vi "Array processor.vi"(10 "Source array":bool[][](array[boolean]), 11 "Pixel size":dbl=12.19 step=0.01) -> (0 "Lenght array":dbl[][](array[numeric]), 3 "T/F product array":bool[][](array[boolean]))   [LabVIEW 2016]
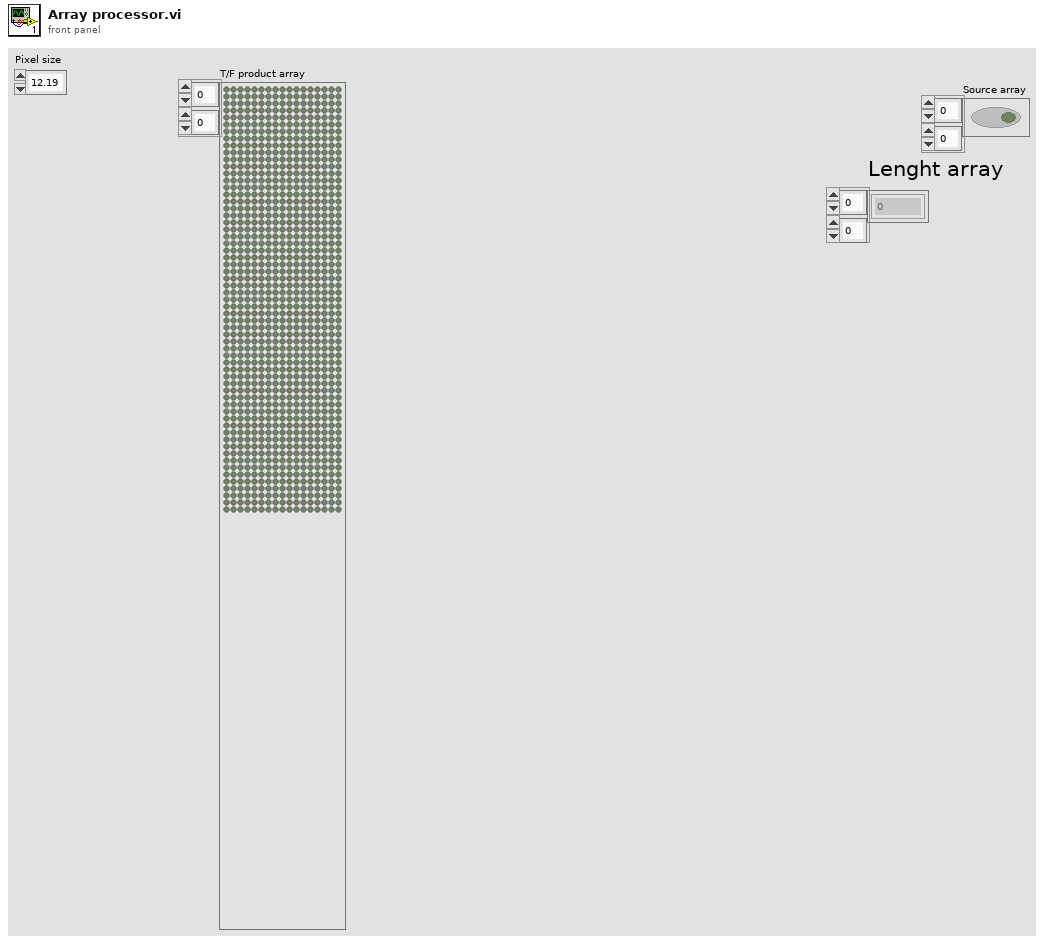
[diagram p1: front panel]
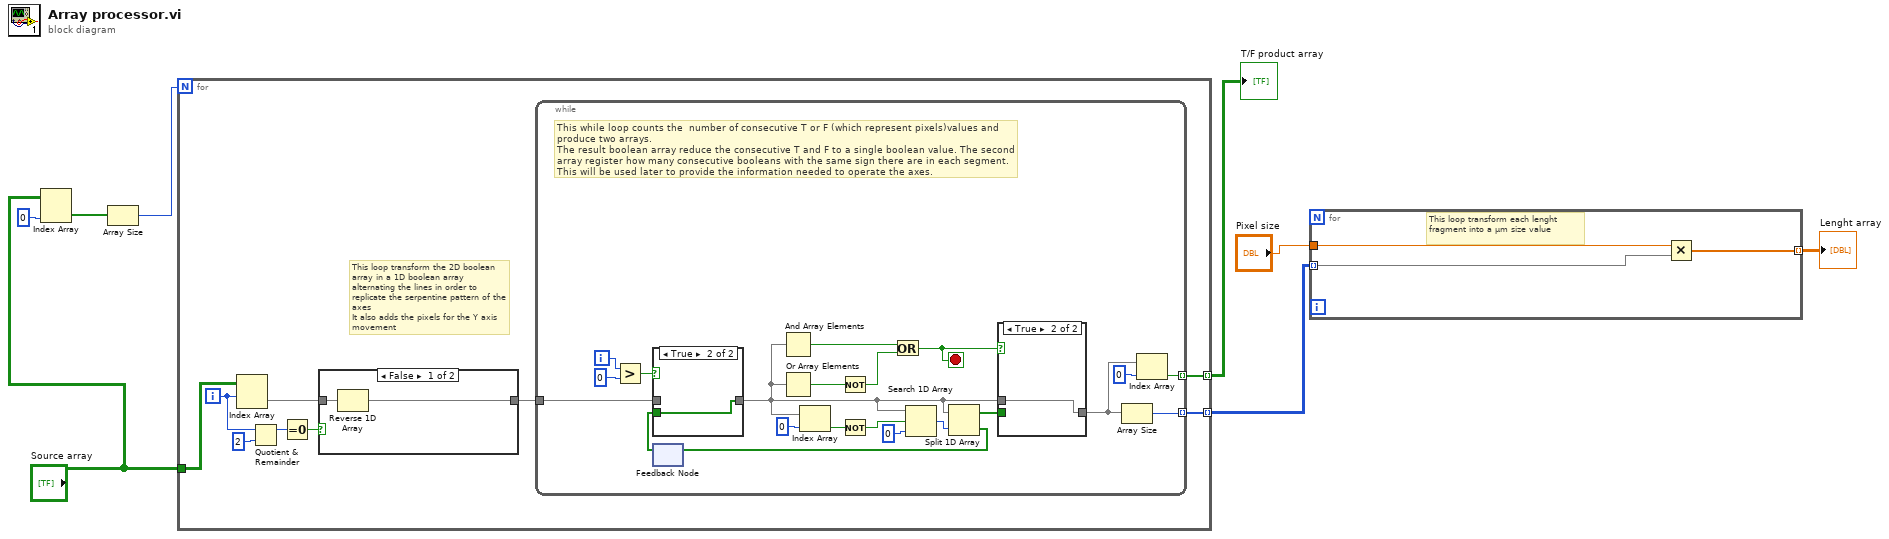
[diagram p0: block diagram]
diagram:
  n1 = Index Array(array="Source array", index (col)=0 ("disabled index (col)")) -> (element=w6:bool[])  [unwired: 1 in]
  n2 = Array Size(array=w6) -> (size(s)=w4:i32)
  n3 = for {
    N: w4 -> [_]
    tunnel: "Source array" -> [w12]
    tunnel: [w10] -> w3 mode=indexing
    tunnel: [w9] -> w8 mode=indexing
    i -> [w15]
    # "This loop transform the 2D boolean array in a 1D boolean array alternating the lines in order to replicate the serpentine pattern of the axes\nIt also adds the pixels for the Y axis movement"
    n4 = Index Array(array=w12, index (row)=w15) -> (element=w13:bool[])  [unwired: 1 in]
    n5 = Quotient & Remainder(x=w15, y=2) -> (x-y*floor(x/y)=w17:i32)  [unwired: 1 out]
    n6 = Equal To 0?(x=w17) -> (x = 0?=w14:bool)
    n7 = case shown="False" w14 {
      tunnel: w13 -> [w44 w45]
      tunnel: [w43 w45] -> w11
      frame False {
        n8 = Reverse 1D Array(array=w44) -> (reversed array=w43:bool[])
      }
      frame True {
      }
    }
    n9 = while {
      tunnel: w11 -> [w32]
      tunnel: [w37] -> w10 mode=indexing
      tunnel: [w18] -> w9 mode=indexing
      i -> [w29]
      stop <- w21 stop-if-true
      # "This while loop counts the  number of consecutive T or F (which represent pixels)values and produce two arrays.\nThe result boolean array reduce the consecutive T and F to a single boolean value. The second array register how many consecutive booleans with the same sign there are in each segment. This will be used later to provide the information needed to operate the axes."
      n10 = Greater?(x=w29, y=0) -> (0:w30:bool)
      n11 = feedback #1() -> (w31:bool[])  [unwired: 1 in]
      n12 = case shown="True" w30 {
        tunnel: w32 -> [w41 _]
        tunnel: [w41 w42] -> w22
        tunnel: w31 -> [_ w42]
        frame False {
        }
        frame True {
        }
      }
      n13 = And Array Elements(Boolean array=w22) -> (logical AND=w26:bool)
      n14 = Or Array Elements(Boolean array=w22) -> (logical OR=w24:bool)
      n15 = Index Array(array=w22, index=0) -> (element=w35:bool)
      n16 = Not(x=w24) -> (.not. x?=w23:bool)
      n17 = Not(x=w35) -> (.not. x?=w34:bool)
      n18 = Or(x=w26, y=w23) -> (x .or. y?=w21:bool)
      n19 = Search 1D Array(1D array=w22, element=w34, start index (0)=0) -> (index of element=w33:i32)
      n20 = Split 1D Array(array=w22, index=w33) -> (first subarray=w25:bool[], second subarray=w27:bool[])
      n21 = feedback-in #1(w27) -> ()
      n22 = case shown="True" w21 {
        tunnel: w25 -> [w39 _]
        tunnel: [w39 w40] -> w20
        tunnel: w22 -> [_ w40]
        frame False {
        }
        frame True {
        }
      }
      n23 = Array Size(array=w20) -> (size(s)=w37:i32)
      n24 = Index Array(array=w20, index=0) -> (element=w18:bool)
    }
  }
  "T/F product array" <- w8
  n25 = for {
    tunnel: w3 -> [w48] mode=indexing
    tunnel: [w47] -> w1 mode=indexing
    tunnel: "Pixel size" -> [w46]
    # "This loop transform each lenght fragment into a µm size value"
    n26 = Multiply(x=w46, y=w48) -> (x*y=w47:dbl[])
  }
  "Lenght array" <- w1
